vi "edittest sequence record to template.vi"(4 "User":T3, 5 "REFQUERY (none)":T2, 6 "Test Station (F)":bool, 7 "POST (empty)":T2, 8 "error in (no error)":errorcluster, 9 "Settings":T1, 10 "Sequence Record (empty)":T5, 11 "Connection Refnum":T4) -> (0 "error out":errorcluster, 1 "Template Keys":T2, 3 "Connection Refnum":T4)   [LabVIEW 2011]
uses:
  server/database/Sequences/Sequence Record.ctl
  ITK EXT/utils/keyedarr.llb/Keyed Array.ctl
  Summitek EXT/ODBC/SQL Controls/Connection Refnum.ctl
  server/database/Users/User Record.ctl
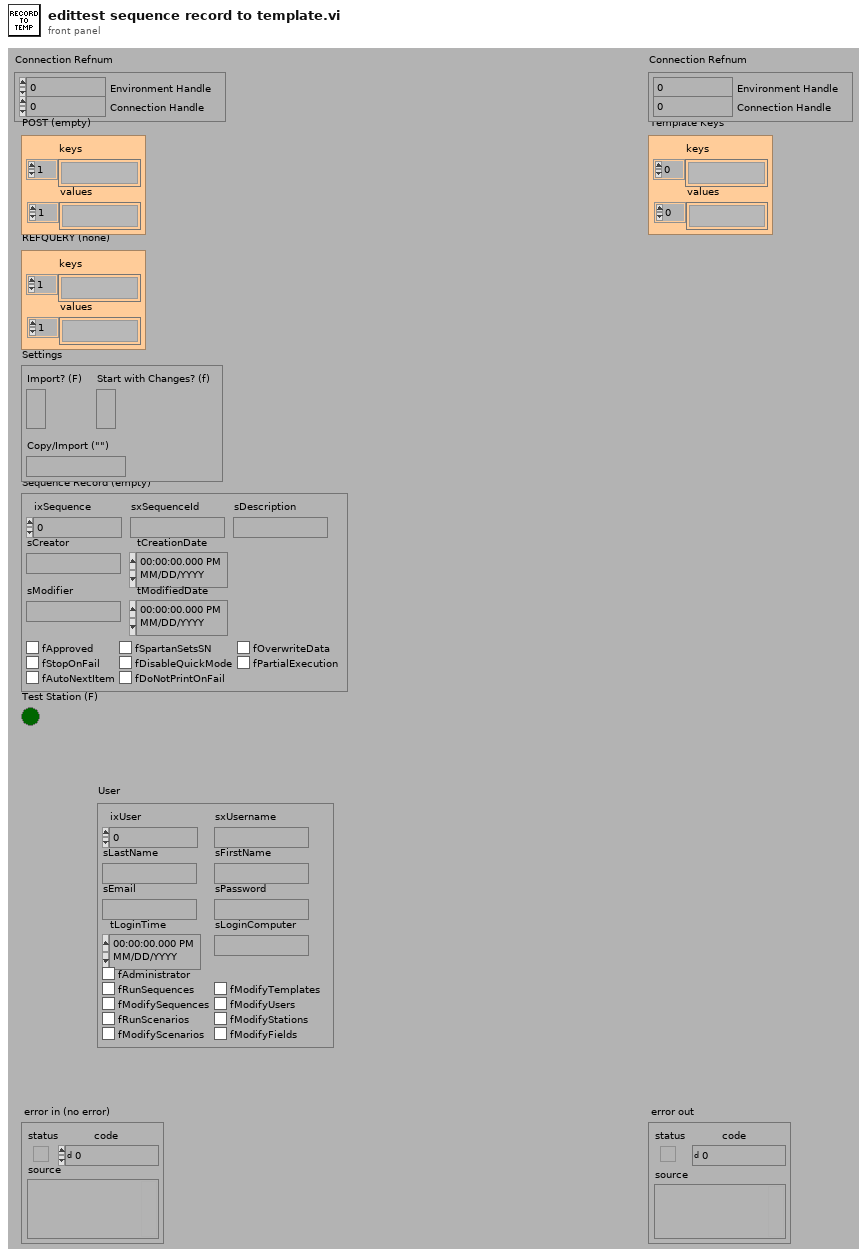
[diagram p1: front panel]
types:
  T1 = cluster{"Import? (F)":bool, "Start with Changes? (f)":bool, "Copy/Import (\"\")":string}
  T2 = typedef "Keyed Array.ctl" = cluster{"keys":string[], "values":string[]}
  T3 = typedef "User Record.ctl" = cluster{"ixUser":i32, "sxUsername":string, "sLastName":string, "sFirstName":string, "sEmail":string, "sPassword":string, "tLoginTime":timestamp, "sLoginComputer":string, "fAdministrator":bool, "fRunSequences":bool, "fModifySequences":bool, "fRunScenarios":bool, "fModifyScenarios":bool, "fModifyTemplates":bool, "fModifyUsers":bool, "fModifyStations":bool, "fModifyFields":bool}
  T4 = typedef "Connection Refnum.ctl" = cluster{"Environment Handle":i32, "Connection Handle":i32}
  T5 = typedef "Sequence Record.ctl" = cluster{"ixSequence":i32, "sxSequenceId":string, "sDescription":string, "sCreator":string, "tCreationDate":timestamp, "sModifier":string, "tModifiedDate":timestamp, "fApproved":bool, "fSpartanSetsSN":bool, "fOverwriteData":bool, "fStopOnFail":bool, "fDisableQuickMode":bool, "fPartialExecution":bool, "fAutoNextItem":bool, "fDoNotPrintOnFail":bool}
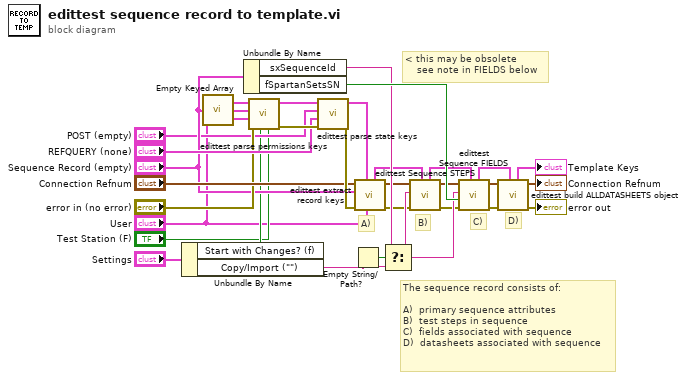
[diagram p0: block diagram]
diagram:
  # "D)"
  # "C)"
  # "B)"
  # "A)"
  # "The sequence record consists of:\n\nA)  primary sequence attributes\nB)  test steps in sequence\nC)  fields associated with sequence\nD)  datasheets associated with sequence"
  # "< this may be obsolete\n    see note in FIELDS below"
  n1 = Unbundle By Name("Settings") -> ("Start with Changes? (f)"=w7:bool, "Copy/Import (\"\")"=w6:string)
  n2 = call "Empty Keyed Array.vi"() -> ("empty keyed array"=w29:T2)  [unwired: 3 out]
  n3 = Unbundle By Name("Sequence Record (empty)") -> ("sxSequenceId"=w22:string, "fSpartanSetsSN"=w23:bool)
  n4 = call "edittest parse permissions keys.vi"("Test Station (F)"="Test Station (F)", "Start with Changes? (f)"=w7, "error in (no error)"="error in (no error)", "User Record"="User", "Sequence Record"="Sequence Record (empty)", "Template Keys In (empty)"=w29) -> ("error out"=w27:errorcluster, "Template Keys Out"=w28:T2)  [unwired: 4 out]
  n5 = call "edittest parse state keys.vi"("error in (no error)"=w27, "REFQUERY (empty)"="REFQUERY (none)", "POST (empty)"="POST (empty)", "Template Keys In (empty)"=w28) -> ("error out"=w25:errorcluster, "Template Keys Out"=w24:T2)  [unwired: 6 out]
  n6 = Empty String/Path?(string/path=w6) -> (empty?=w1:bool)
  n7 = call "edittest extract record keys.vi"("User Record"="User", "Template Keys In (empty)"=w24, "error in (no error)"=w25, "Sequence Record"="Sequence Record (empty)", "Connection Refnum"="Connection Refnum") -> ("error out"=w15:errorcluster, "Connection Refnum"=w16:T4, "Template Keys Out"=w14:T2)  [unwired: 4 out]
  n8 = Select(t=w22, s=w1, f=w6) -> (s? t:f=w21:string)
  n9 = call "edittest Sequence STEPS.vi"("Template Keys In (empty)"=w14, "error in (no error)"=w15, "Sequence Id (\"\")"=w21, "Connection Refnum"=w16) -> ("error out"=w10:errorcluster, "Connection Refnum"=w13:T4, "Template Keys Out"=w12:T2)  [unwired: 3 in, 2 out]
  n10 = call "edittest Sequence FIELDS.vi"("Template Keys In (empty)"=w12, "error in (no error)"=w10, "fSpartanSetsSN"=w23, "Sequence Id (\"\")"=w21, "Connection Refnum"=w13) -> ("error out"=w4:errorcluster, "Connection Refnum"=w9:T4, "Template Keys Out"=w11:T2)  [unwired: 2 in, 2 out]
  n11 = call "edittest build ALLDATASHEETS object.vi"("Template (empty)"=w11, "error in (no error)"=w4, "Connection Refnum"=w9) -> ("error out"=→"error out":errorcluster, "Connection Refnum"=→"Connection Refnum":T4, "new Template"=→"Template Keys":T2)  [unwired: 1 in, 5 out]
